vi "T2 Tests.vi"() -> ()   [LabVIEW 2014]
panel:
  in  "#Repetitions":i32
  in  "stop":bool
  in  "?":enum32{"T2", "Rabi"}(tab)
  in  "Pi time":dbl[](array[slide]) scale=0.0..10.0
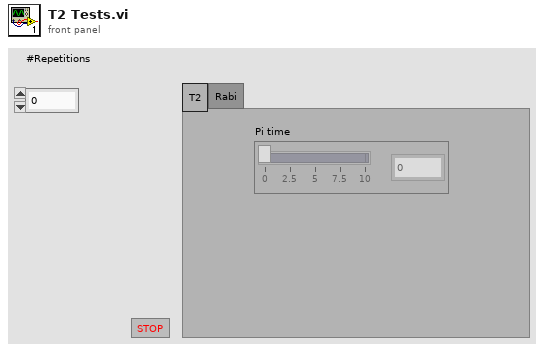
[diagram p1: front panel]
types:
  T1 = cluster{"Pi_time":dbl[], "Pulse_width_us":dbl, "MW_width_us":dbl, "Dark_times_us":dbl[], "Sampling mode":enum16{"Normal", "Sweep"}, "#Pi_pulses":i32, "Repetitions":i32}
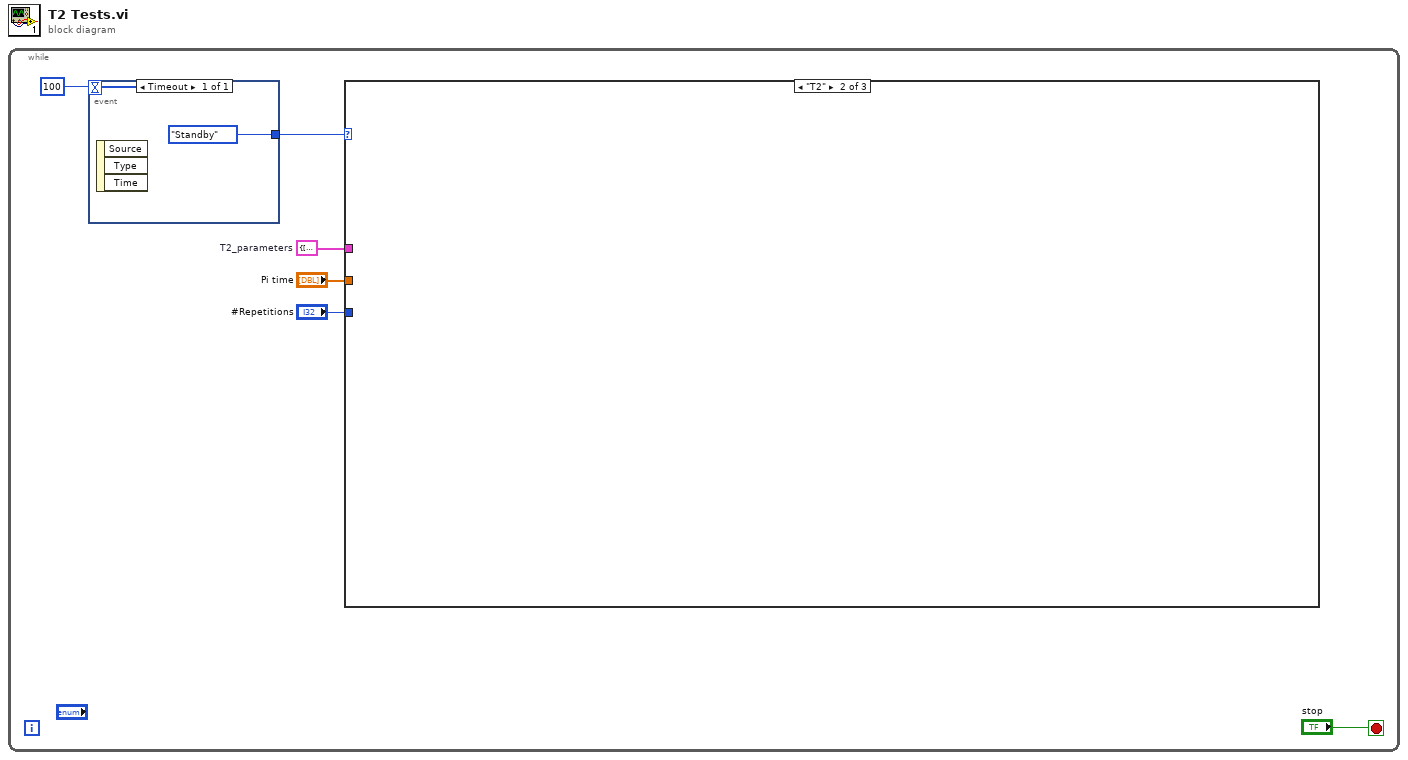
[diagram p0: block diagram]
diagram:
  n1 = while {
    stop <- "stop" stop-if-true
    w3 = T1 {"Pi_time"=[], "Pulse_width_us"=0.0, "MW_width_us"=0.0, "Dark_times_us"=[], "Sampling mode"=enum."Normal", "#Pi_pulses"=0, "Repetitions"=0}  # T2_parameters
    n2 = event shown="[0] Timeout" {
      selector: _ -> [_]
      dyn-events: _ -> [_]
      timeout: 100 -> [_]
      tunnel: [enum16{"Standby", "T2", "Rabi"}."Standby"] -> w4
      event Timeout {
        n3 = event-data() -> ()  [unwired: 1 in, 3 out]
      }
    }
    n4 = case shown="\"T2\"" w4 {
      tunnel: w3 -> [_ _ _]
      tunnel: "Pi time" -> [_ _ _]
      tunnel: "#Repetitions" -> [_ _ _]
      frame "Standby", Default {
      }
      frame "T2" {
      }
      frame "Rabi" {
      }
    }
  }
